vi "DS18x20 Temperature Sensor.vi"   [LabVIEW 2014]
doc: "Test VI for template library."
uses:
  QwaveSys_Interface/QwaveSys_Interface.lvlib
  QwaveSys_ESP8266/QwaveSys_ESP8266.lvlib
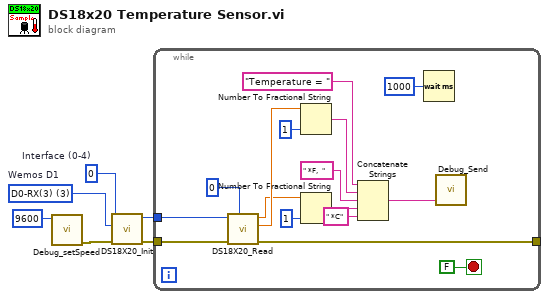
[diagram p0: block diagram]
diagram:
  w2 = u8 3 items=["D0-RX(3)"=3, "D1-TX(1)"=1, "D2(16)"=16, "D3/D15/SCL(5)"=5, "D4/D14/SDA(4)"=4, "D5/D13/SCK(14)-(LED)"=14, "D6/D12/MISO(12)"=12, "D7/D11/MOSI(13)"=13, "D8(0)"=0, "D9/TX1(2)"=2, "D10/SS (15)"=15, "ADC0,(17)"=17]  # Wemos D1
  w4 = u8 0  # Interface (0-4)
  n1 = call "Debug_setSpeed.vi"("Speed"=u32 9600) -> ("error out"=w3:errorcluster)  [unwired: 10 in]
  n2 = call "DS18X20_Init.vi"("error in"=w3, "PIN"=w2, "Interface (0-4)"=w4) -> ("error out"=w6:errorcluster, "Instance"=w5:u8)  [unwired: 7 in]
  n3 = while {
    tunnel: w6 -> [w22]
    tunnel: w5 -> [w10]
    tunnel: [w7] -> _
    stop <- FALSE stop-if-true
    n4 = call "DS18X20_Read.vi"("Index"=i8 0, "error in (no error)"=w22, "Instance"=w10) -> ("error out"=w7:errorcluster, "F"=w16:dbl, "C"=w15:dbl)  [unwired: 6 in]
    n5 = Number To Fractional String(number=w16, precision (6)=i16 1) -> (F-format string=w20:string)  [unwired: 2 in]
    n6 = Number To Fractional String(number=w15, precision (6)=i16 1) -> (F-format string=w19:string)  [unwired: 2 in]
    n7 = Concatenate Strings("Temperature = " ("format string"), w20, " *F,  " ("format string"), w19, " *C" ("string")) -> (w8:string)
    n8 = Wait (ms)(milliseconds to wait=u32 1000) -> ()  [unwired: 1 out]
    n9 = call "Debug_Send.vi"("DATA"=w8) -> ()  [unwired: 11 in]
  }
